vi "Reset Acquisition.vi"(8 "error in":errorcluster, 11 "eCRDS in":refnum<class "eCRDS.lvclass">) -> (0 "error out":errorcluster, 3 "eCRDS out":refnum<class "eCRDS.lvclass">)   [LabVIEW 2014, in "eCRDS Library.lvlib" / "eCRDS.lvclass"]
uses:
  eCRDS.lvclass
  eCRDS.lvclass/eCRDS.ctl
  <vilib>/DAQmx/read.llb/DAQmx Read (Analog 2D DBL NChan NSamp).vi
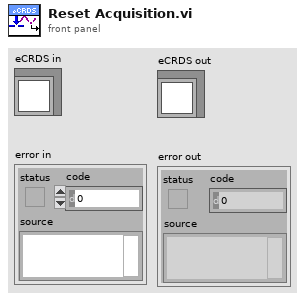
[diagram p1: front panel]
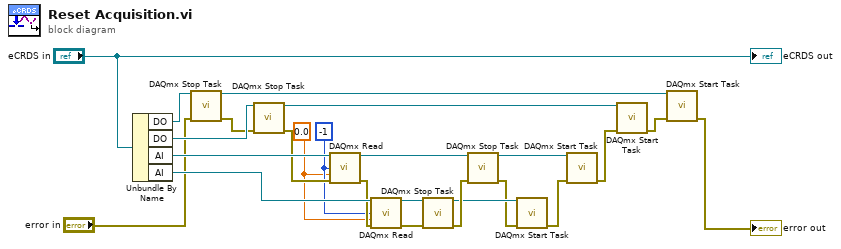
[diagram p0: block diagram]
diagram:
  w5 = 0.0 ("timeout")
  w6 = -1 ("number of samples per channel")
  n1 = Unbundle By Name("eCRDS in") -> ("DO"=w19:refnum<k21>, "DO"=w18:refnum<k21>, "AI"=w12:refnum<k21>, "AI"=w9:refnum<k21>)
  n2 = call <vilib>:"DAQmx Stop Task.vi"("task/channels in"=w19, "error in"="error in") -> ("task out"=w13:refnum<k21>, "error out"=w17:errorcluster)  [unwired: 12 in]
  n3 = call <vilib>:"DAQmx Stop Task.vi"("task/channels in"=w18, "error in"=w17) -> ("task out"=w16:refnum<k21>, "error out"=w10:errorcluster)  [unwired: 12 in]
  n4 = call-poly <vilib>:"DAQmx Read.vi"("task/channels in"=w12, "number of samples per channel"=w6, "timeout"=w5, "error in"=w10) -> ("task out"=w11:refnum<k21>, "error out"=w7:errorcluster)  [unwired: 9 in, 1 out]
  n5 = call-poly <vilib>:"DAQmx Read.vi"("task/channels in"=w9, "number of samples per channel"=w6, "timeout"=w5, "error in"=w7) -> ("task out"=w8:refnum<k21>, "error out"=w4:errorcluster)  [unwired: 9 in, 1 out]
  n6 = call <vilib>:"DAQmx Stop Task.vi"("task/channels in"=w8, "error in"=w4) -> ("task out"=w23:refnum<k21>, "error out"=w24:errorcluster)  [unwired: 12 in]
  n7 = call <vilib>:"DAQmx Stop Task.vi"("task/channels in"=w11, "error in"=w24) -> ("task out"=w20:refnum<k21>, "error out"=w22:errorcluster)  [unwired: 12 in]
  n8 = call <vilib>:"DAQmx Start Task.vi"("task/channels in"=w23, "error in"=w22) -> ("error out"=w21:errorcluster)  [unwired: 12 in, 1 out]
  n9 = call <vilib>:"DAQmx Start Task.vi"("task/channels in"=w20, "error in"=w21) -> ("error out"=w15:errorcluster)  [unwired: 12 in, 1 out]
  n10 = call <vilib>:"DAQmx Start Task.vi"("task/channels in"=w16, "error in"=w15) -> ("error out"=w14:errorcluster)  [unwired: 12 in, 1 out]
  n11 = call <vilib>:"DAQmx Start Task.vi"("task/channels in"=w13, "error in"=w14) -> ("error out"=→"error out":errorcluster)  [unwired: 12 in, 1 out]
  "eCRDS out" <- "eCRDS in"
